vi "Read Input Registers.vi"(8 "error in (no error)":errorcluster, 9 "number of registers":u16, 10 "starting address":u16, 11 "device data model in":refnum<class "Standard Data Model.lvclass">) -> (0 "error out":errorcluster, 2 "data":u16[](array[numeric]), 3 "device data model out":refnum<class "Standard Data Model.lvclass">)   [LabVIEW 2020, in "SubVIs.lvlib" / "Standard Data Model.lvclass"]
doc: "Reads N input registers from the device model, starting at register M."
uses:
  <vilib>/Modbus/subvis/Data and Functions/Standard Data Model/Standard Data Model.lvclass
  <vilib>/Modbus/subvis/Data and Functions/Standard Data Model/Standard Data Model.lvclass/Standard Data Model.ctl
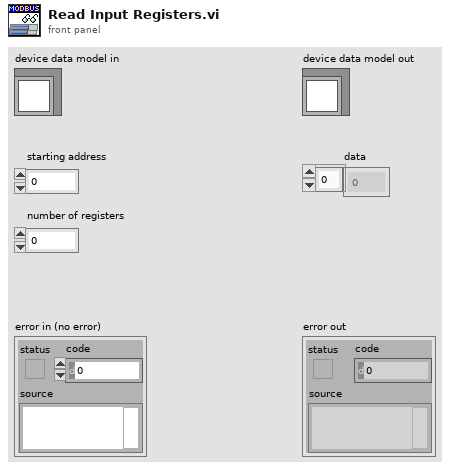
[diagram p1: front panel]
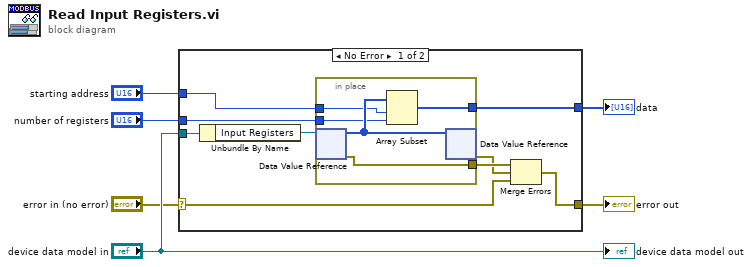
[diagram p0: block diagram]
diagram:
  n1 = case shown="No Error" "error in (no error)" {
    selector: "error in (no error)" -> [w7 w21]
    tunnel: "device data model in" -> [w15 _]
    tunnel: [w14 _] -> w5
    tunnel: "starting address" -> [w12 _]
    tunnel: "number of registers" -> [w11 _]
    tunnel: [w10 w21] -> w2
    frame No Error {
      n2 = Unbundle By Name(w15) -> ("Input Registers"=w13:refnum<data-value>)
      n3 = in-place {
        in-place-border: [w19] -> w14
        in-place-border: w12 -> [w18]
        in-place-border: w11 -> [w17]
        in-place-border: [w16] -> w9
        n4 = in-place-dvr #1(w13) -> (w20:u16[], w16:errorcluster)
        n5 = Array Subset(array=w20, index=w18, length=w17) -> (w19:u16[])
        n6 = in-place-dvr #1(w20) -> (w8:errorcluster)  [unwired: 1 out]
      }
      n7 = Merge Errors(w9, w8, w7) -> (w10:errorcluster)
    }
    frame Error {
    }
  }
  "error out" <- w2
  "data" <- w5
  "device data model out" <- "device data model in"
